vi "Control_Channel_Status.vi"() -> ()   [LabVIEW 2010]
uses:
  Sub VIs/ADAM Controls/Channel_State.ctl
  Sub VIs/ADAM Controls/Channel_names.ctl
  Anemometry/Anemometry Sub Vis/Globals/Preference_global.vi
panel:
  out "Turn On?":bool
  in  "Turn Channel Off?":bool
  in  "stop":bool
  out "Ch State":T1
  in  "Turn Channels On?":bool
  in  "Selected Channels to Edit":i32[](listbox)
  in  "Search Charcters":string
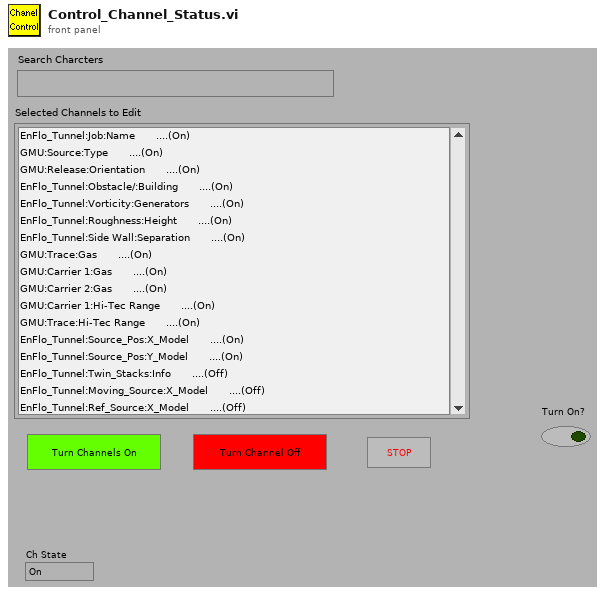
[diagram p1: front panel]
types:
  T1 = typedef "Channel_State.ctl" = enum16{"On", "Off", "Always On", "Always Off"}
  T2 = typedef "Channel_names.ctl" = enum16{"Active Only", "Active + Off", "All Channels"}
  T3 = typedef "Server_Comms.ctl" = enum16{"Server Link Healthy", "Do Not Link To Server"}
  T4 = typedef "Ch_description_ADAM.ctl" = cluster{"Ch Name":string, "Type":T5, "Function":T6, "Ch State":T1, "Calibration type":T7, "A":dbl, "B":dbl, "C":dbl, "D":dbl, "Comments":string, "Address":T8, "String":string, "Duty":u16}
  T5 = typedef "Module_type_ADAM.ctl" = enum16{"4011", "4012", "4013", "4014", "4016", "4017", "4018", "4021", "4050", "4052", "4053", "4060", "4080", "5000", "5017", "5018", "5024", "5051", "5056", "5060", "6060", "Tracker", "WEST", "GILL", "JEM", "VICI", "Vaisala", "DRUCK", "Run VI Named:", "IR2100", "PPT", "Comparator", "VIRTUAL", "Hold Value", "Read A", "Read Ch", "Coded", "Client Info", "Web Client", "X10", "Test"}
  T6 = typedef "Function_ADAM.ctl" = enum16{"Analogue Input", "Digital Input", "Event counter", "Event rate", "Analogue Output", "Digital Output", "Relay Output"}
  T7 = typedef "Calib_type_ADAM.ctl" = enum16{"Raw", "Bx + A", "Cx^2 + Bx + A", "Dx^3 + Cx^2 + Bx + A", "In Band", "Hi-Tec Q", "Hi-Tec M_dot", "Text"}
  T8 = typedef "Address.ctl" = cluster{"Main":i32, "Ch.":i32, "Sub":i32, "Port Name":string}
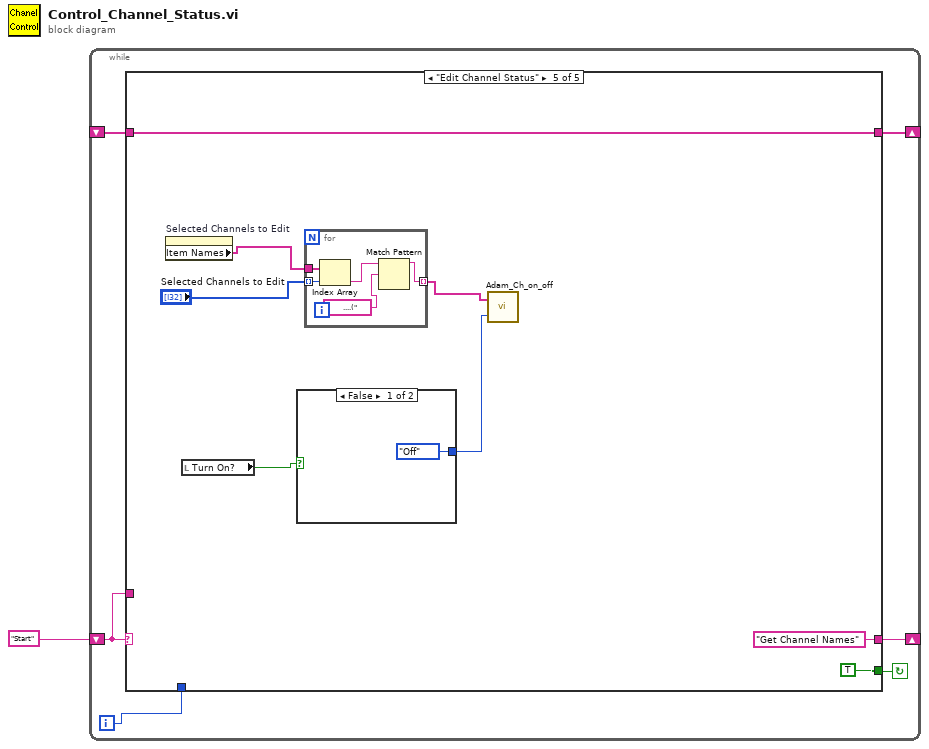
[diagram p0: block diagram]
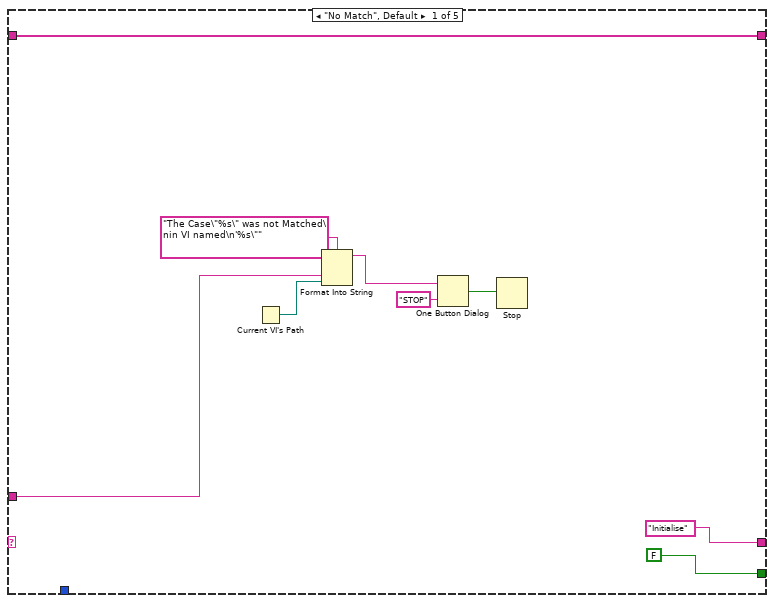
[diagram p2: hidden frame]
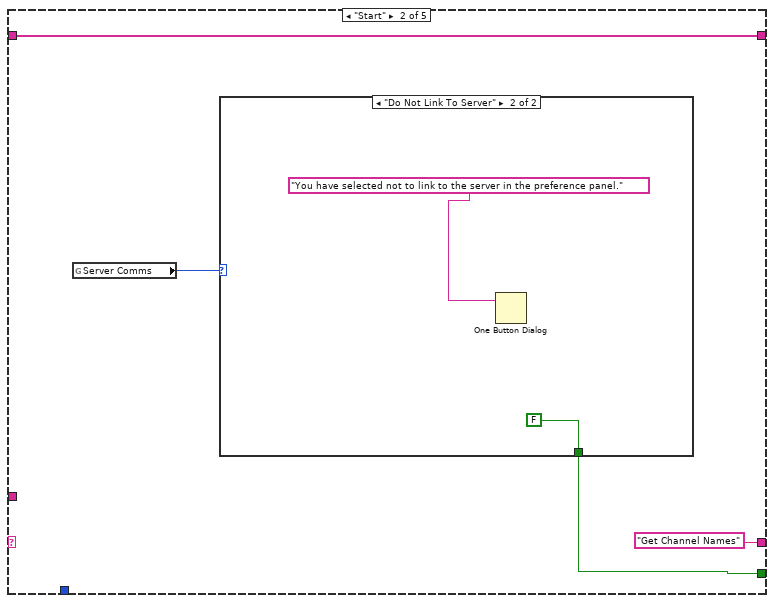
[diagram p3: hidden frame]
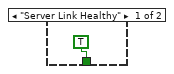
[diagram p4: hidden frame]
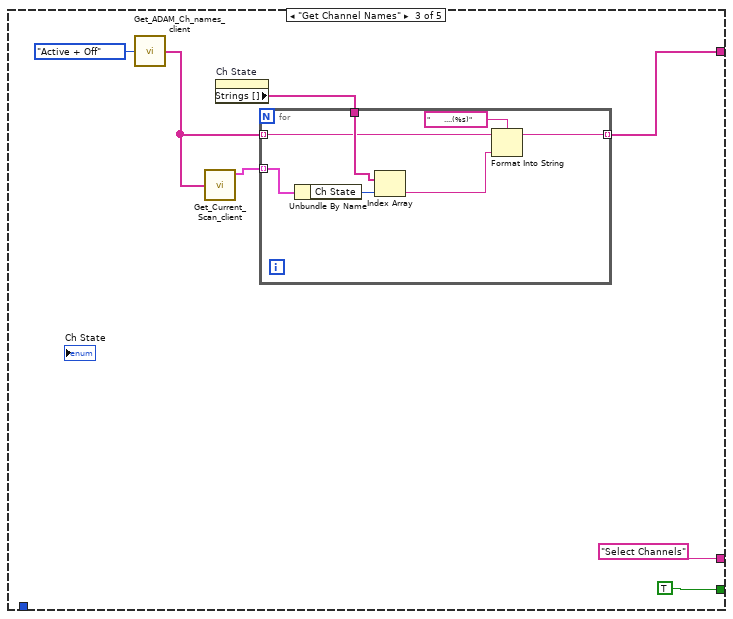
[diagram p5: hidden frame]
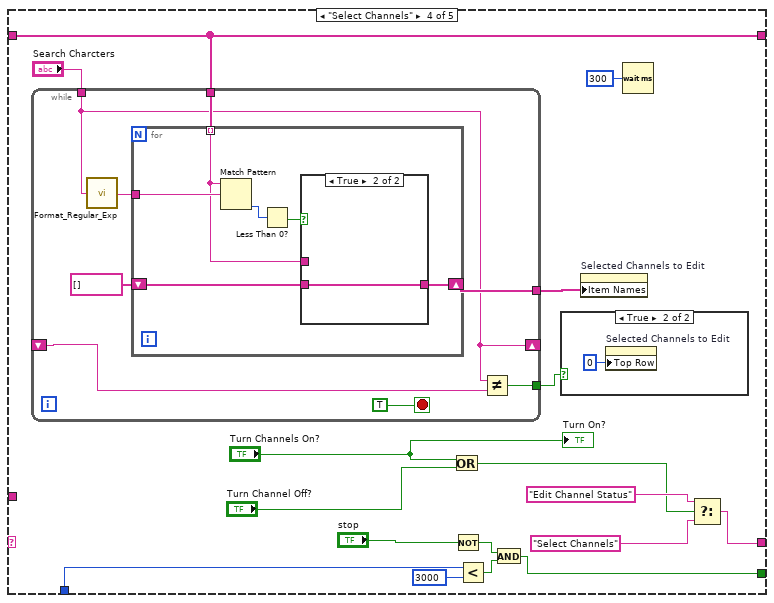
[diagram p6: hidden frame]
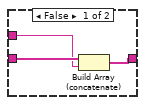
[diagram p8: hidden frame]
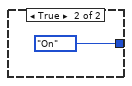
[diagram p9: hidden frame]
diagram:
  n1 = while {
    shift-left: "Start" -> [w5]
    shift-right: [w6] -> _
    shift-right: [w4] -> _
    shift-left: _ -> [w3]
    i -> [w2]
    stop <- w7 continue-if-true
    n2 = case shown="\"Edit Channel Status\"" w5 {
      tunnel: [FALSE w18 TRUE w41 TRUE] -> w7
      tunnel: ["Initialise" "Get Channel Names" "Select Channels" w51 "Get Channel Names"] -> w6
      tunnel: w5 -> [w11 _ _ _ _]
      tunnel: [w8 w17 w24 w49 w81] -> w4
      tunnel: w3 -> [w8 w17 _ w49 w81]
      tunnel: w2 -> [_ _ _ w40 _]
      frame "No Match", Default {
        n3 = Current VI's Path() -> (path=w10:path)
        n4 = Format Into String(format string="The Case\"%s\" was not Matched\nin VI named\n'%s\"" ("Format String"), w11, w10) -> (resulting string=w14:string)  [unwired: 2 in, 1 out]
        n5 = One Button Dialog(message=w14, button name ("OK")="STOP") -> (true=w12:bool)
        n6 = Stop(stop? (T)=w12) -> ()
      }
      frame "Start" {
        n7 = global read "Preference_global.vi" "Server Comms"() -> (w19:T3)
        n8 = case shown="\"Do Not Link To Server\"" w19 {
          tunnel: [TRUE FALSE] -> w18
          frame "Server Link Healthy" {
          }
          frame "Do Not Link To Server" {
            n9 = One Button Dialog(message="You have selected not to link to the server in the preference panel.") -> ()  [unwired: 2 out]
          }
        }
      }
      frame "Get Channel Names" {
        n10 = call "Get_ADAM_Ch_names_client.vi"("Channel names set"=Channel_names."Active + Off") -> ("Ch names"=w25:string[])
        n11 = call "Get_Current_Scan_client.vi"("ADAM Ch Names"=w25) -> ("Ch Description Array"=w27:T4[])  [unwired: 3 out]
        n12 = property on="Ch State" class="Enum (strict)"() -> ("Strings []"=w26:string[])  [unwired: 2 in, 2 out]
        n13 = for {
          tunnel: w27 -> [w37] mode=indexing
          tunnel: w26 -> [w36]
          tunnel: w25 -> [w34] mode=indexing
          tunnel: [w31] -> w24 mode=indexing
          n14 = Unbundle By Name(w37) -> ("Ch State"=w35:T1)
          n15 = Index Array(array=w36, index=w35) -> (element=w33:string)
          n16 = Format Into String(format string="       ....(%s)", initial string=w34, w33) -> (resulting string=w31:string)  [unwired: 1 in, 1 out]
        }
      }
      frame "Select Channels" {
        n17 = while {
          tunnel: [w62] -> w54
          tunnel: w49 -> [w61]
          tunnel: "Search Charcters" -> [w59]
          shift-right: [w59] -> _
          shift-left: _ -> [w58]
          tunnel: [w57] -> w38
          stop <- TRUE stop-if-true
          n18 = call "Format_Regular_Exp.vi"("Regular expression"=w59) -> ("Case Insensitive for html"=w60:string)
          n19 = for {
            tunnel: w60 -> [w69]
            shift-right: [w65] -> w62
            shift-left: string[] [] -> [w66]
            tunnel: w61 -> [w64] mode=indexing
            n20 = Match Pattern(string=w64, regular expression=w69) -> (offset past match=w68:i32)  [unwired: 4 out]
            n21 = Less Than 0?(x=w68) -> (x < 0?=w67:bool)
            n22 = case shown="True" w67 {
              tunnel: w66 -> [w72 w73]
              tunnel: [w71 w73] -> w65
              tunnel: w64 -> [w70 _]
              frame False {
                n23 = Build Array (concatenate)(w72, w70) -> (w71:string[])
              }
              frame True {
              }
            }
          }
          n24 = Not Equal?(x=w59, y=w58) -> (x != y?=w57:bool)
        }
        n25 = Or(x="Turn Channels On?", y="Turn Channel Off?") -> (x .or. y?=w44:bool)
        n26 = Not(x="stop") -> (.not. x?=w43:bool)
        n27 = Less?(x=w40, y=3000) -> (x < y?=w42:bool)
        n28 = And(x=w43, y=w42) -> (x .and. y?=w41:bool)
        n29 = case shown="True" w38 {
          frame False {
          }
          frame True {
            n30 = property on="Selected Channels to Edit" class="LstBox (strict)"("Top Row"=0) -> ()  [unwired: 2 in, 2 out]
          }
        }
        n31 = property on="Selected Channels to Edit" class="LstBox (strict)"("Item Names"=w54) -> ()  [unwired: 2 in, 2 out]
        n32 = Wait (ms)(milliseconds to wait=u32 300) -> ()  [unwired: 1 out]
        n33 = Select(t="Edit Channel Status", s=w44, f="Select Channels") -> (s? t:f=w51:string)
        "Turn On?" <- "Turn Channels On?"
      }
      frame "Edit Channel Status" {
        n34 = property on="Selected Channels to Edit" class="LstBox (strict)"() -> ("Item Names"=w77:string[])  [unwired: 2 in, 2 out]
        n35 = local read "Turn On?"() -> (w75:bool)
        n36 = case shown="False" w75 {
          tunnel: [Channel_State."Off" ("Ch State") Channel_State."On" ("Ch State")] -> w74
          frame False {
          }
          frame True {
          }
        }
        n37 = for {
          tunnel: "Selected Channels to Edit" -> [w88] mode=indexing
          tunnel: w77 -> [w87]
          tunnel: [w86] -> w76 mode=indexing
          n38 = Index Array(array=w87, index=w88) -> (element=w84:string)
          n39 = Match Pattern(string=w84, regular expression="       ....(" ("format string")) -> (before substring=w86:string)  [unwired: 4 out]
        }
        n40 = call "Adam_Ch_on_off.vi"("Ch State"=w74, "ADAM Ch Names"=w76) -> ()  [unwired: 1 out]
      }
    }
  }
